vi "RVC Drive to Line.vi"() -> ()   [LabVIEW 2013]
uses:
  <vilib>/Simulation/Scripting/Companion Diagram/SimConfigNode/SimParams.ctl
  <vilib>/Simulation/Scripting/Companion Diagram/SimConfigNode/_simSolvers.ctl
  <vilib>/Simulation/Implementation/Shared/SIMSCR Execution Mode.ctl
  <vilib>/Simulation/Param Hierarchy/Typedefs/SIMPH Param Control Actions.ctl
  <vilib>/Simulation/Scripting/Editor Utilities/SIM subVI tag data.ctl
  <vilib>/Simulation/Scripting/Editor Utilities/SIM subVI execution type.ctl
  <vilib>/Simulation/Implementation/Shared/NILVSim_ParamChanged.vi
  <vilib>/Simulation/Implementation/Shared/NILVSIM_BeginStep.vi
  <vilib>/Simulation/Utility/Implementation/SIM Time.vi
  <vilib>/Analysis/coordinate.llb/Wrap Angle.vi
  <vilib>/Analysis/coordinate.llb/Wrap Angle (scalar).vi
  <vilib>/Simulation/SignalArithmetic/Implementation/NILVSim Gain.llb/SIM Gain (scalar).vi
  <vilib>/Simulation/Utility/Implementation/SIM Halt.vi
  <vilib>/Simulation/Utility/Implementation/NILVSim Collector.llb/SIM Collector (vector).vi
  <vilib>/Simulation/Implementation/Shared/SIM Fire Discrete SubVI.vi
  <vilib>/Simulation/Implementation/Shared/NILVSim_Manager.vi
  <vilib>/Simulation/Implementation/Shared/NILVSim_FinalizeModel.vi
  <vilib>/Simulation/Utility/Implementation/NILVSim Collector.llb/NILVSim Collector core (vector).vi
  <vilib>/Simulation/Implementation/Shared/SIM Fire Discrete SubVI (Core).vi
  <vilib>/Simulation/Implementation/Shared/SIM Unbundle Sim Info.vi
  <vilib>/Utility/error.llb/Clear Errors.vi
  <vilib>/Simulation/Implementation/Shared/NILVSim_GetModelError.vi
  <vilib>/Simulation/Implementation/Shared/SIM Bundle Sim Info.vi
  <vilib>/Simulation/Implementation/Shared/SIMSH Read Queue.vi
  <vilib>/Simulation/Implementation/Shared/NILVSim_Initialize.vi
  <vilib>/Simulation/Utility/Implementation/NILVSim Get Time and IsAcceptedStep.vi
  subVIs/2D Animate Rotating Wheel.vi
  subVIs/2D Animation.vi
  <vilib>/Simulation/Scripting/Companion Diagram/SimConfigNode/SimDog.xnode
  SIM Bicycle.vi
  <vilib>/Simulation/Implementation/XNodeFramework/SimXNode/SimX.xnode
  <vilib>/Analysis/NI_AAL_Angle.lvlib
  <vilib>/Simulation/Implementation/Shared/NI_SIM_Implementation.lvlib
panel:
  out "velocity":dbl(knob)=1.0 scale=0.0..10.0
  out "XY Graph - Drive to Line":cluster{"Time":dbl[], "Signal":dbl[]}[](graph)
  out "Position":cluster{"x":dbl, "y":dbl, "theta":dbl}
  out "Steering Angle":dbl format="%.2f"
  out "Steering Angle":picture
  out "Map Floor":picture
  # "Velocity"
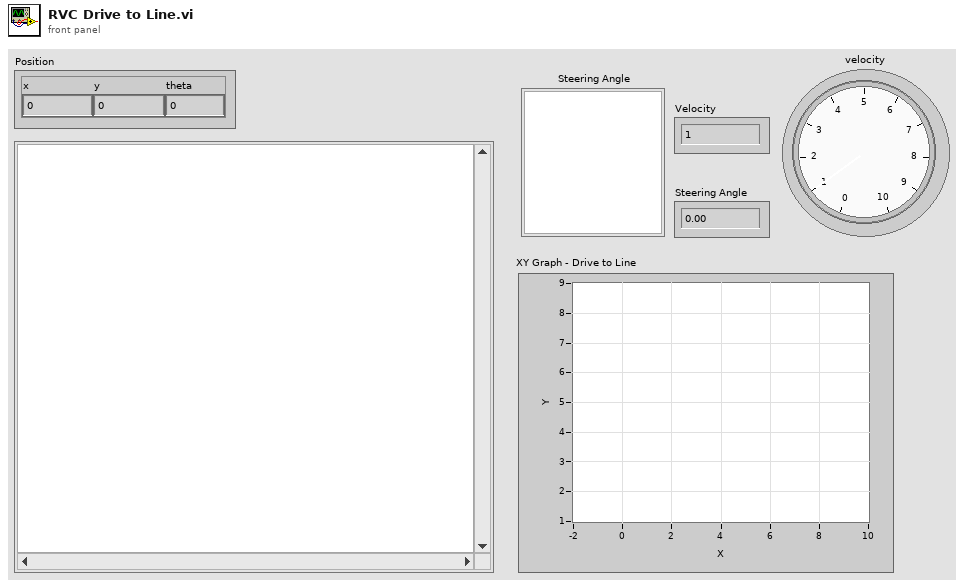
[diagram p1: front panel]
types:
  T1 = typedef "SIMSCR Execution Mode.ctl" = enum16{"Simulate to Completion", "Single Time-Step Simulation (Fixed Step Only)"}
  T2 = typedef "SIMPH Param Control Actions.ctl" = enum16{"get params", "set params"}
  T3 = typedef "SIM subVI tag data.ctl" = cluster{"period":dbl, "skew":dbl, "Simulation execution type":T4}
  T4 = typedef "SIM subVI execution type.ctl" = enum16{"Function call", "Discrete", "Continuous", "Initialization only", "Final step only"}
  T5 = cluster{"SIMSH Sim Time":dbl, "Build Array 2":cluster{"appended array":dbl[]}, "Divide 2":cluster{"x/y":dbl}, "Sine & Cosine":cluster{"sin(x)":dbl, "cos(x)":dbl}, "initial condition":dbl[], "Index Array 4":cluster{"element":dbl}, "vel limit":cluster{"output":dbl}, "steering angle limit":cluster{"output":dbl}, "acceleration limit":cluster{"output":dbl}, "Product":cluster{"Result":dbl[]}, "Build Array":cluster{"appended array":dbl[]}, "Integrator":cluster{"output":dbl[]}}
  T6 = typedef "SimParams.ctl" = cluster{"Initial Time (s)":dbl, "Final Time (s)":dbl, "Step Size (s)":dbl, "ODE Solver":T7, "Minimum Step Size (s)":dbl, "Maximum Step Size (s)":dbl, "Relative Tolerance":dbl, "Absolute Tolerance":dbl, "Software Timing":bool, "Initial Step Size (s)":dbl, "Automatic Fixed Step Size?":bool, "Automatic Discrete Step Size?":bool, "Discrete Step Size (s)":dbl, "Calculate using Time Step":bool, "Solver Wired?":bool, "Prev.Frm.Expected End":u64, "Prev.Frm.Actual End":u64, "Prev.Frm.Finished Late?":bool, "Prev.Iter.Expected End":u64, "Prev.Iter.Actual End":u64, "Prev.Iter.Finished Late?":bool, "Expected Iteration Start":u64, "Actual Iteration Start":u64, "Expected Frame Start":u64, "Actual Frame Start":u64, "Source Name":string, "Name":string, "Period":i64, "Deadline":i64, "Offset":i64, "Start":i64, "Priority":i32, "Timeout":i32, "Processor":i32, "Mode":enum32{"No Change", "Process missed periods, maintain original phase", "Discard missed periods, maintain original phase", "Process missed periods, ignore original phase", "Discard missed periods, ignore original phase"}, "Wakeup reason":enum32{"Normal", "Aborted", "Asynchronous wakeup", "Timing source error", "Timed loop error", "Timeout"}, "Error":errorcluster, "Source Type":string, "Secondary Source Type":string, "Global End Time":u64, "Global Start Time":u64, "Full Solver Reset":bool, "Execution Mode":T1, "Nan/Inf Check":bool, "Custom Solver Library":string, "Solver Is Variable":bool, "custom solver name":string, "Signal Collection Decimation":u32}
  T7 = typedef "_simSolvers.ctl" = enum16{"Runge-Kutta 1 (Euler)", "Runge-Kutta 2", "Runge-Kutta 3", "Runge-Kutta 4", "Runge-Kutta 23 (variable)", "Runge-Kutta 45 (variable)", "BDF (variable)", "Adams-Moulton (variable)", "Rosenbrock (variable)", "Discrete States Only", "SDIRK 4 (variable)", "Radau 5 (variable)", "Radau 9 (variable)", "Radau 13 (variable)", "Radau [Variable Order] (variable)", "Gear's Method (variable)", "Linearizer", "State Query", "Trim Eval", "Custom Solver"}
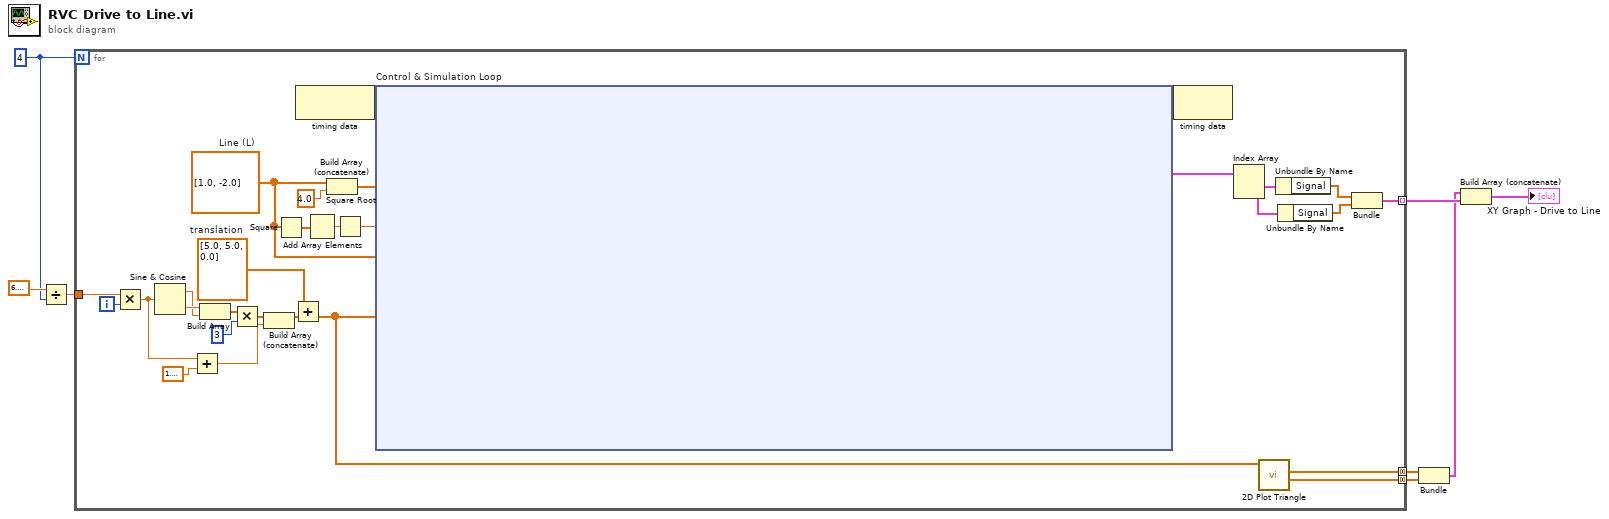
[diagram p0: block diagram]
diagram:
  w6 = 4
  n1 = Divide(x=6.283185307179586, y=w6) -> (x/y=w5:dbl)
  n2 = for {
    N: w6 -> [_]
    tunnel: [w28] -> w8 mode=indexing
    tunnel: w5 -> [w24]
    tunnel: [w19] -> w3 mode=concatenating
    tunnel: [w18] -> w2 mode=concatenating
    i -> [w25]
    w12 = dbl[] [1.0, -2.0]  # Line (L)
    w15 = dbl[] [5.0, 5.0, 0.0]  # translation
    n3 = Multiply(x=w24, y=w25) -> (x*y=w20:dbl)
    n4 = Sine & Cosine(0:w20) -> (1:w26:dbl, 2:w27:dbl)
    n5 = Add(x=w20, y=1.5707963267948966) -> (x+y=w17:dbl)
    n6 = Build Array(w27, w26) -> (w35:dbl[])
    n7 = Multiply(x=w35, y=3) -> (x*y=w34:dbl[])
    n8 = Build Array (concatenate)(w34, w17) -> (w21:dbl[])
    n9 = Square(x=w12) -> (x^2=w10:dbl[])
    n10 = Add(x=w15, y=w21) -> (x+y=w16:dbl[])
    n11 = node-c288() -> (w37:variant)  [unwired: 1 in]
    n12 = Add Array Elements(numeric array=w10) -> (sum=w11:dbl)
    n13 = Build Array (concatenate)(w12, 4.0) -> (w14:dbl[])
    n14 = Square Root(x=w11) -> (sqrt(x)=w9:dbl)
    n15 = node-c254 "Control & Simulation Loop"(w37, w16, w12, w14, w9) -> (w36:variant, w33:cluster{"Time":dbl[], "Signal":dbl[]}[])
    n16 = node-c288(w36) -> ()  [unwired: 1 out]
    n17 = Index Array(array=w33) -> (element #1=w32:cluster{"Time":dbl[], "Signal":dbl[]}, element #2=w31:cluster{"Time":dbl[], "Signal":dbl[]})  [unwired: 2 in]
    n18 = call "2D Plot Triangle.vi"("appended array"=w16) -> ("Y"=w18:dbl[], "X"=w19:dbl[])  [unwired: 8 in, 1 out]
    n19 = Unbundle By Name(w32) -> ("Signal"=w30:dbl[])
    n20 = Unbundle By Name(w31) -> ("Signal"=w29:dbl[])
    n21 = Bundle("Signal"=w30, "Signal"=w29) -> (w28:cluster{"Signal":dbl[], "Signal":dbl[]})  [unwired: 1 in]
  }
  n22 = Bundle("X"=w3, "Y"=w2) -> (w1:cluster{"X":dbl[], "Y":dbl[]})  [unwired: 1 in]
  n23 = Build Array (concatenate)(w1, w8) -> (→"XY Graph - Drive to Line":cluster{"Signal":dbl[], "Signal":dbl[]}[])
